vi "S8300E_BARCODE_SN_MAC.vi"() -> ()   [LabVIEW 2011]
uses:
  <vilib>/event_ctls.llb/eventvkey.ctl
panel:
  out "軟體版本Software Version":string
  out "begin":u32
  in  "Product SN產品序號":string="192.168.1.3\n192.168.1.1\n192.168.1.1"
  in  "LAN MAC":string="192.168.1.3\n192.168.1.1\n192.168.1.1"
  # "輸入條碼上的資訊"
  # "2015-1-8"
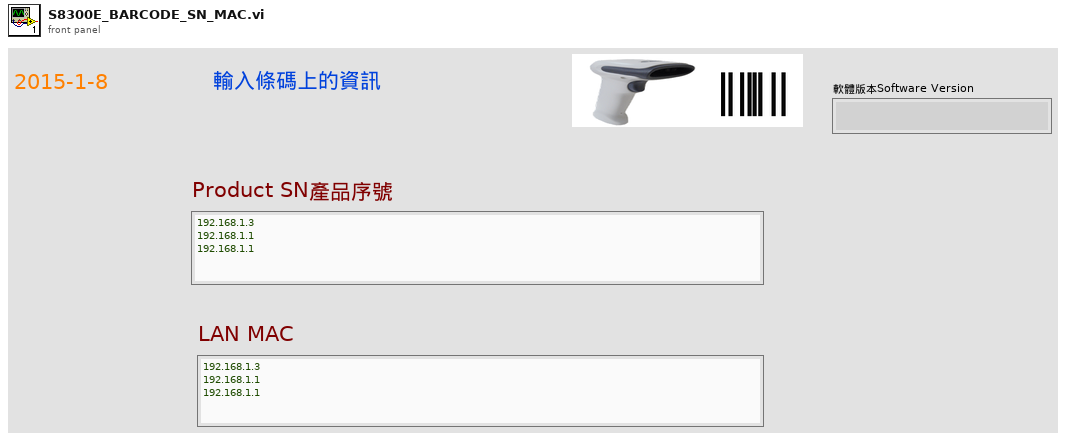
[diagram p1: front panel]
types:
  T1 = typedef "eventvkey.ctl" = enum16{"ASCII", "Enter", "Return", "Shift", "Ctrl", "Alt", "Cmd", "Opt", "Caps", "NumLock", "Clear", "Break", "Up", "Down", "Left", "Right", "Insert", "Delete", "Home", "End", "PageUp", "PageDown", "Escape", "Help", "Pause", "ScrollLock", "F1", "F2", "F3", "F4", "F5", "F6", "F7", "F8", "F9", "F10", "F11", "F12", "F13", "F14", "F15", "F16", "F17", "F18", "F19", "F20", "F21", "F22", "F23", "F24", "Play", "VolumeUp", "VolumeDown", "Mute", "Two Byte Char"}
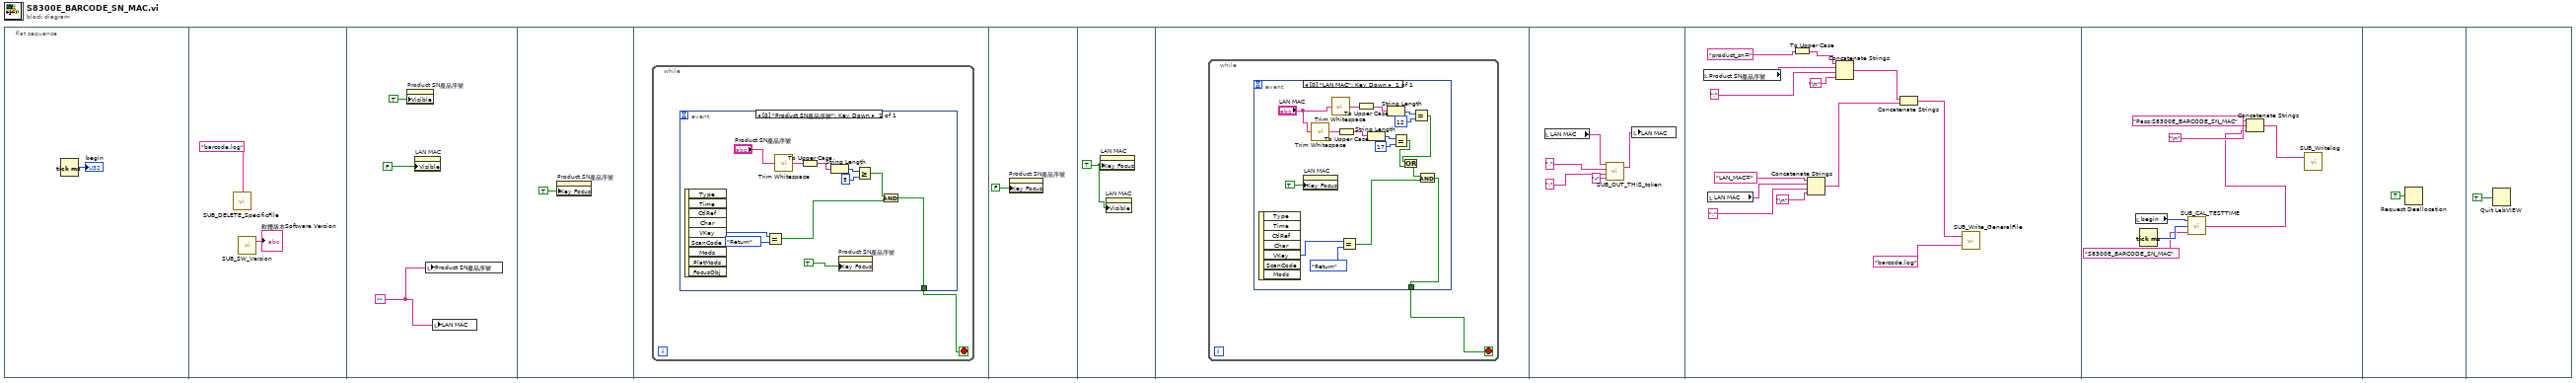
[diagram p0: block diagram]
diagram:
  n1 = flat-sequence {
    frame #0 {
      n2 = Tick Count (ms)() -> (millisecond timer value=→"begin":u32)
    }
    frame #1 {
      n3 = call "SUB_DELETE_SpecificFile.vi"("Filename to be  Deleted"="barcode.log" ("Filename")) -> ()  [unwired: 2 in, 1 out]
      n4 = call "SUB_SW_Version.vi"() -> ("Current Software Version"=→"軟體版本Software Version":string)  [unwired: 3 in]
    }
    frame #2 {
      w4 = ""
      n5 = property on="Product SN產品序號" class="Str"("Visible"=TRUE) -> ()  [unwired: 2 in, 2 out]
      n6 = property on="LAN MAC" class="Str"("Visible"=FALSE) -> ()  [unwired: 2 in, 2 out]
      n7 = local write "Product SN產品序號"(w4) -> ()
      n8 = local write "LAN MAC"(w4) -> ()
    }
    frame #3 {
      n9 = property on="Product SN產品序號" class="Str"("Key Focus"=TRUE) -> ()  [unwired: 2 in, 2 out]
    }
    frame #4 {
      n10 = while {
        stop <- w8 stop-if-true
        n11 = event shown="[0] \"Product SN產品序號\": Key Down" {
          selector: _ -> [_]
          dyn-events: _ -> [_]
          timeout: _ -> [_]
          tunnel: [w10] -> w8
          event "Product SN產品序號": Key Down {
            n12 = event-data() -> ("VKey"=w13:T1)  [unwired: 1 in, 8 out]
            n13 = Equal?(x=w13, y=eventvkey."Return") -> (x = y?=w11:bool)
            n14 = call <vilib>:"Trim Whitespace.vi"("string"="Product SN產品序號") -> ("trimmed string"=w16:string)  [unwired: 1 in]
            n15 = To Upper Case(1:w16) -> (0:w15:string)
            n16 = String Length(string=w15) -> (length=w19:i32)
            n17 = property on="Product SN產品序號" class="Str"("Key Focus"=TRUE) -> ()  [unwired: 2 in, 2 out]
            n18 = Greater Or Equal?(x=w19, y=5) -> (x >= y?=w17:bool)
            n19 = And(x=w17, y=w11) -> (x .and. y?=w10:bool)
          }
        }
      }
    }
    frame #5 {
      n20 = property on="Product SN產品序號" class="Str"("Key Focus"=FALSE) -> ()  [unwired: 2 in, 2 out]
    }
    frame #6 {
      w21 = TRUE ("Key Focus")
      n21 = property on="LAN MAC" class="Str"("Key Focus"=w21) -> ()  [unwired: 2 in, 2 out]
      n22 = property on="LAN MAC" class="Str"("Visible"=w21) -> ()  [unwired: 2 in, 2 out]
    }
    frame #7 {
      n23 = while {
        stop <- w22 stop-if-true
        n24 = event shown="[0] \"LAN MAC\": Key Down" {
          selector: _ -> [_]
          dyn-events: _ -> [_]
          timeout: _ -> [_]
          tunnel: [w35] -> w22
          event "LAN MAC": Key Down {
            n25 = event-data() -> ("VKey"=w39:T1)  [unwired: 1 in, 6 out]
            n26 = property on="LAN MAC" class="Str"("Key Focus"=TRUE) -> ()  [unwired: 2 in, 2 out]
            n27 = call <vilib>:"Trim Whitespace.vi"("string"="LAN MAC") -> ("trimmed string"=w28:string)  [unwired: 1 in]
            n28 = call <vilib>:"Trim Whitespace.vi"("string"="LAN MAC") -> ("trimmed string"=w33:string)  [unwired: 1 in]
            n29 = To Upper Case(1:w28) -> (0:w27:string)
            n30 = Equal?(x=w39, y=eventvkey."Return") -> (x = y?=w34:bool)
            n31 = To Upper Case(1:w33) -> (0:w32:string)
            n32 = String Length(string=w27) -> (length=w30:i32)
            n33 = String Length(string=w32) -> (length=w37:i32)
            n34 = Equal?(x=w30, y=17) -> (x = y?=w23:bool)
            n35 = Equal?(x=w37, y=12) -> (x = y?=w24:bool)
            n36 = Or(x=w24, y=w23) -> (x .or. y?=w25:bool)
            n37 = And(x=w25, y=w34) -> (x .and. y?=w35:bool)
          }
        }
      }
    }
    frame #8 {
      n38 = local read "LAN MAC"() -> (w44:string)
      n39 = call "SUB_OUT_THIS_token.vi"("Remove token symbl1 3"="-", "Remove token symbl1 2"=":" ("Remove token symbl1"), "Remove token symbl1"=".", "input string"=w44) -> ("result string"=w40:string)  [unwired: 1 in]
      n40 = local write "LAN MAC"(w40) -> ()
    }
    frame #9 {
      n41 = local read "Product SN產品序號"() -> (w56:string)
      n42 = local read "LAN MAC"() -> (w53:string)
      n43 = To Upper Case(1:"product_sn=" ("string")) -> (0:w45:string)
      n44 = Concatenate Strings("LAN_MAC=" ("string"), w53, ";", "\n") -> (w50:string)
      n45 = Concatenate Strings(w45, w56, ";", "\n") -> (w51:string)
      n46 = Concatenate Strings(w51, w50) -> (w49:string)
      n47 = call "SUB_Write_GeneralFile.vi"("Filename"="barcode.log", "Text Input"=w49) -> ()  [unwired: 1 out]
    }
    frame #10 {
      n48 = local read "begin"() -> (w64:u32)
      n49 = Tick Count (ms)() -> (millisecond timer value=w63:u32)
      n50 = call "SUB_CAL_TESTTIME.vi"("Test Item name"="S8300E_BARCODE_SN_MAC", "Stop tick time"=w63, "Start tick time"=w64) -> ("Test Time output"=w59:string)  [unwired: 2 in]
      n51 = Concatenate Strings("Pass:S8300E_BARCODE_SN_MAC" ("string"), "\n", w59) -> (w58:string)
      n52 = call "SUB_Writelog.vi"("Pass/Fail"=w58) -> ()  [unwired: 2 in]
    }
    frame #11 {
      n53 = Request Deallocation(TRUE ("flag")) -> ()
    }
    frame #12 {
      n54 = Quit LabVIEW(quit? (T)=TRUE) -> ()
    }
  }
